vi "DetectChange.vi"(11 "Value":i32) -> (3 "Changed":bool)   [LabVIEW 2023]
doc: "Returns true if the value changed"
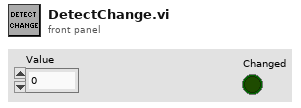
[diagram p1: front panel]
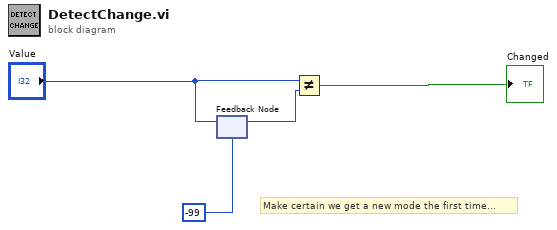
[diagram p0: block diagram]
diagram:
  # "Make certain we get a new mode the first time..."
  n1 = feedback-in #1("Value") -> ()
  n2 = feedback #1(-99 ("Value")) -> (w4:i32)
  n3 = Not Equal?(x="Value", y=w4) -> (x != y?=→"Changed":bool)
